vi "XY- Graph As Chart.vi"(2 "Clear Graph (F)":bool, 3 "Maxi Points (10,000)":dbl=10000.0, 4 "Y-Value":dbl, 5 "X- Value":dbl) -> (1 "XY Graph":cluster{dbl[], dbl[]}(graph))   [LabVIEW 2011]
doc: "This vi takes in a X-Value and a Y-Value and adds those values into two arrays and formats the data to go into an XY-Graph inside of a while loop. This causes the XY-Graph to behave as a chart. \n\n- Place this VI in a while loop, along with an XY-Graph\n- Wire in a dynamic X-Value, and a dynamic Y-Value\n- Wire out to the XY-Graph\n- Hit Run on your Main VI\n- You can limit the number of data points in the graph by wiring in a numeric value (default is 10,000)\n- You can clear the values in the graph before each run by wiring in the stop boolean to this VI"
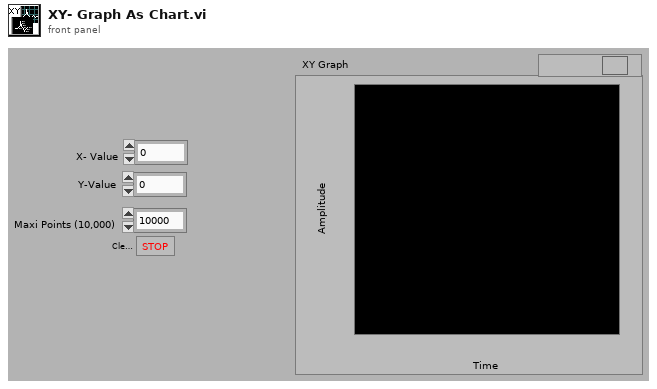
[diagram p1: front panel]
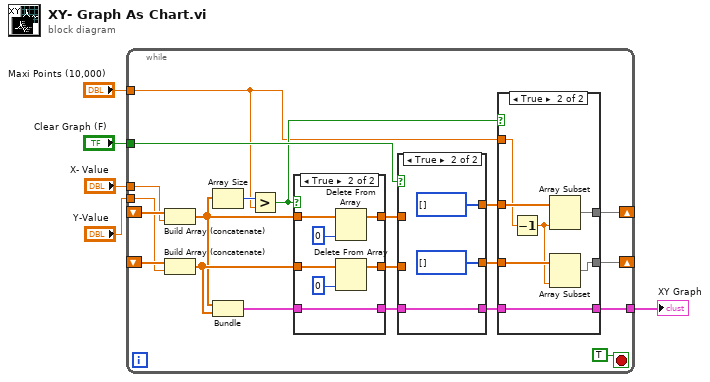
[diagram p0: block diagram]
diagram:
  n1 = while {
    shift-right: [w10] -> _
    shift-left: _ -> [w23]
    tunnel: "Clear Graph (F)" -> [w19]
    tunnel: "X- Value" -> [w16]
    tunnel: "Y-Value" -> [w15]
    tunnel: [w9] -> w2
    shift-right: [w12] -> _
    shift-left: _ -> [w22]
    tunnel: "Maxi Points (10,000)" -> [w6]
    stop <- TRUE stop-if-true
    n2 = Build Array (concatenate)(w22, w16) -> (w25:dbl[])
    n3 = Build Array (concatenate)(w23, w15) -> (w26:dbl[])
    n4 = Array Size(array=w25) -> (size(s)=w24:i32)
    n5 = Bundle(w25, w26) -> (w20:cluster{dbl[], dbl[]})  [unwired: 1 out]
    n6 = Greater?(x=w24, y=w6) -> (0:w7:bool)
    n7 = case shown="True" w7 {
      tunnel: w26 -> [w44 w50]
      tunnel: w25 -> [w45 w48]
      tunnel: [w44 w49] -> w17
      tunnel: [w45 w47] -> w18
      tunnel: w20 -> [w43 w46]
      tunnel: [w43 w46] -> w14
      frame False {
      }
      frame True {
        n8 = Delete From Array(array=w48, index=0) -> (array with subset deleted=w47:dbl[])  [unwired: 1 in, 1 out]
        n9 = Delete From Array(array=w50, index=0) -> (array with subset deleted=w49:dbl[])  [unwired: 1 in, 1 out]
      }
    }
    n10 = case shown="True" w19 {
      tunnel: [w38 i32[] []] -> w11
      tunnel: [w39 i32[] []] -> w13
      tunnel: w18 -> [w39 _]
      tunnel: w17 -> [w38 _]
      tunnel: w14 -> [w37 w40]
      tunnel: [w37 w40] -> w8
      frame False {
      }
      frame True {
      }
    }
    n11 = case shown="True" w7 {
      tunnel: w13 -> [w29 w36]
      tunnel: [w29 w34] -> w12
      tunnel: w11 -> [w28 w35]
      tunnel: [w28 w33] -> w10
      tunnel: [w27 w31] -> w9
      tunnel: w8 -> [w27 w31]
      tunnel: w6 -> [_ w30]
      frame False {
      }
      frame True {
        n12 = Decrement(x=w30) -> (x-1=w32:dbl)
        n13 = Array Subset(array=w36, length=w32) -> (w34:dbl[])  [unwired: 1 in]
        n14 = Array Subset(array=w35, length=w32) -> (w33:dbl[])  [unwired: 1 in]
      }
    }
  }
  "XY Graph" <- w2
